vi "Filter.vi"(0 "VisaCluster":T1, 7 "Filter":bool, 11 "error in (no error)":errorcluster) -> (4 "VisaCluster":T1, 6 "Filter 2":bool, 8 "Answer":string, 10 "Display":string, 15 "error out":errorcluster)   [LabVIEW 2014, in "FH 55.lvlib"]
doc: "This VI sets the Filter ON or OFF. \n\nDurch das VI Filter kann die Funktion an und ausgeschaltet werden. Die Funktion Filter wird verwendet, um eine ruhigere Anzeige des Messwertes zu erzielen. Die Funktion ist so ausgelegt, dass langsam veränderliche Felder dargestellt werden und das Rauschen unterdrückt wird."
uses:
  FH 55.lvlib
  TypeDef/VisaCluster.ctl
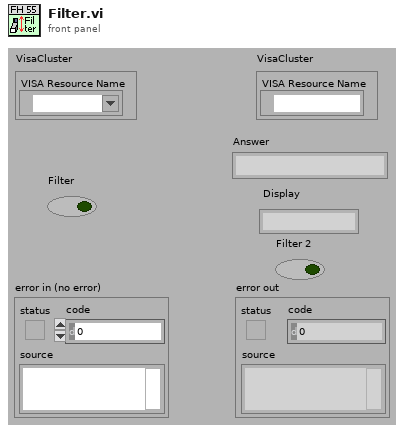
[diagram p1: front panel]
types:
  T1 = typedef "FH 55.lvlib/VisaCluster.ctl" = cluster{"VISA Resource Name":refnum<visa-resource-name>}
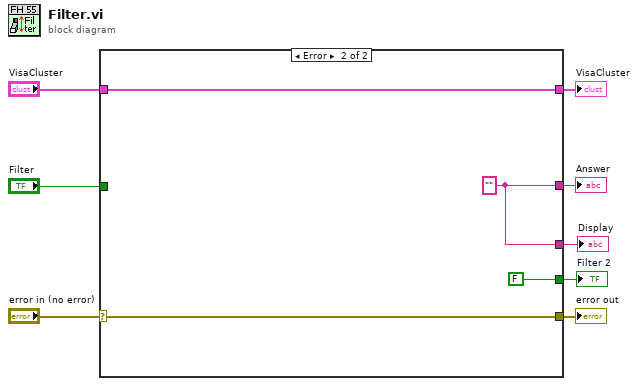
[diagram p0: block diagram]
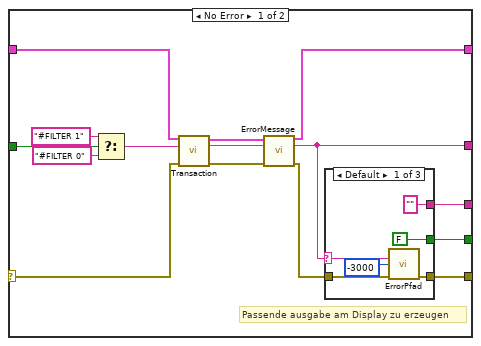
[diagram p2: hidden frame]
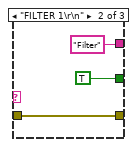
[diagram p3: hidden frame]
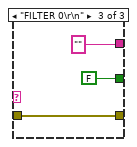
[diagram p4: hidden frame]
diagram:
  n1 = case shown="Error" "error in (no error)" {
    selector: "error in (no error)" -> [w17 w38]
    tunnel: "VisaCluster" -> [w19 w39]
    tunnel: "Filter" -> [w23 _]
    tunnel: [w20 w39] -> w4
    tunnel: [w11 w38] -> w6
    tunnel: [w13 w37] -> w5
    tunnel: [w12 w37] -> w2
    tunnel: [w9 FALSE] -> w1
    frame No Error {
      # "Passende ausgabe am Display zu erzeugen"
      n2 = Select(t="#FILTER 1", s=w23, f="#FILTER 0") -> (s? t:f=w18:string)
      n3 = call "Transaction.vi"("VisaCluster"=w19, "Command"=w18, "error in (no error)"=w17) -> ("VisaCluster"=w14:T1, "Answer"=w15:string, "error out"=w16:errorcluster)  [unwired: 9 in, 1 out]
      n4 = call "ErrorMessage.vi"("VisaCluster"=w14, "Message In"=w15, "error in (no error)"=w16) -> ("VisaCluster"=w20:T1, "Message Out"=w13:string, "error out"=w10:errorcluster)  [unwired: 10 in]
      n5 = case shown="Default" w13 {
        selector: w13 -> [w26 _ _]
        tunnel: ["" "Filter" ""] -> w12
        tunnel: [w28 w31 w34] -> w11
        tunnel: w10 -> [w27 w31 w34]
        tunnel: [FALSE TRUE FALSE] -> w9
        frame Default {
          n6 = call "ErrorPfad.vi"("Message In"=w26, "Numeric"=-3000, "error in (no error)"=w27) -> ("error out"=w28:errorcluster)  [unwired: 11 in, 1 out]
        }
        frame "FILTER 1\r\n" {
        }
        frame "FILTER 0\r\n" {
        }
      }
    }
    frame Error {
      w37 = ""
    }
  }
  "error out" <- w6
  "Answer" <- w5
  "VisaCluster" <- w4
  "Display" <- w2
  "Filter 2" <- w1
